vi "Day 1.vi"(11 "Input File":enum32{"example input", "input"}(radio)) -> (3 "sum":i16)   [LabVIEW 2021]
uses:
  <vilib>/Utility/file.llb/Read Delimited Spreadsheet (I64).vi
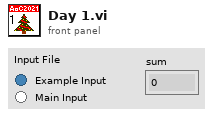
[diagram p1: front panel]
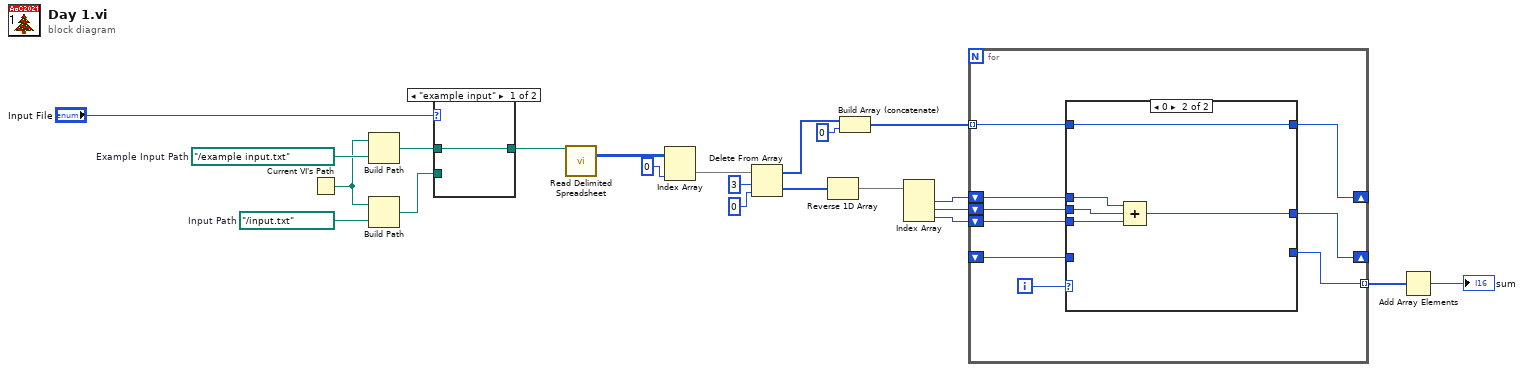
[diagram p0: block diagram]
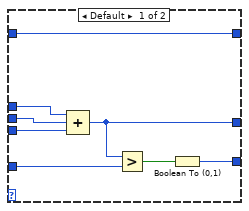
[diagram p2: hidden frame]
diagram:
  w21 = path "../example input.txt"  # Example Input Path
  w22 = path "../input.txt"  # Input Path
  n1 = Current VI's Path() -> (path=w14:path)
  n2 = Build Path(base path=w14, name or relative path=w21) -> (appended path=w18:path)
  n3 = Build Path(base path=w14, name or relative path=w22) -> (appended path=w19:path)
  n4 = case shown="\"example input\"" "Input File" {
    tunnel: w19 -> [_ w24]
    tunnel: w18 -> [w23 _]
    tunnel: [w23 w24] -> w17
    frame "example input" {
    }
    frame "input" {
    }
  }
  n5 = call-poly <vilib>:"Read Delimited Spreadsheet.vi"("file path (dialog if empty)"=w17) -> ("all rows"=w16:i64[][])  [unwired: 9 in, 5 out]
  n6 = Index Array(array=w16, index (col)=0 ("disabled index (col)")) -> (element=w11:i64[])  [unwired: 1 in]
  n7 = Delete From Array(array=w11, length=3, index=0) -> (deleted portion=w5:i64[], array with subset deleted=w8:i64[])
  n8 = Reverse 1D Array(array=w5) -> (reversed array=w1:i64[])
  n9 = Build Array (concatenate)(w8, 0) -> (w10:i64[])
  n10 = Index Array(array=w1) -> (element #1=w3:i64, element #2=w4:i64, element #3=w2:i64)  [unwired: 3 in]
  n11 = for {
    tunnel: w10 -> [w32] mode=indexing
    shift-right: [w31] -> _
    shift-left: w3 -> [w30]
    tunnel: [w29] -> w13 mode=indexing
    shift-left: w4 -> [w28]
    shift-left: w2 -> [w27]
    shift-right: [w26] -> _
    shift-left: _ -> [w25]
    i -> [w33]
    n12 = case shown="0" w33 {
      tunnel: w32 -> [w38 w44]
      tunnel: [w38 w44] -> w31
      tunnel: w30 -> [w37 w46]
      tunnel: [w40 _] -> w29
      tunnel: w28 -> [w36 w45]
      tunnel: w27 -> [w35 w43]
      tunnel: [w34 w42] -> w26
      tunnel: w25 -> [w39 _]
      frame Default {
        n13 = Compound Arithmetic op=ADD(w37, w36, w35) -> (w34:i64)
        n14 = Greater?(x=w34, y=w39) -> (0:w41:bool)
        n15 = Boolean To (0,1)(Boolean=w41) -> (0, 1=w40:i16)
      }
      frame 0 {
        n16 = Compound Arithmetic op=ADD(w46, w45, w43) -> (w42:i64)
      }
    }
  }
  n17 = Add Array Elements(numeric array=w13) -> (sum=→"sum":i16)
